vi "ni579x Configure Attenuation.vi"(0 "Register Bus":refnum<class "ni579x Register Bus v1 Host.lvclass">=refnum, 1 "scope":string(combo)="rx/atten1", 5 "attenuation [dB]":dbl format="%#_6p", 11 "Error In":errorcluster) -> (4 "Register Bus (out)":refnum<class "ni579x Register Bus v1 Host.lvclass">, 6 "coerced attenuation [dB]":dbl format="%#_6p", 15 "Error Out":errorcluster)   [LabVIEW 2013]
uses:
  <instrlib>/ni579x/Register Bus/v1/Host/ni579x Register Bus v1 Host.lvclass
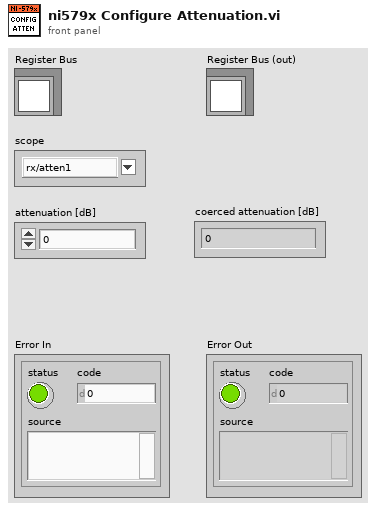
[diagram p1: front panel]
types:
  T1 = typedef "ni579x User Command.ctl" = cluster{"User Data 0":u8, "User Data 1":u8, "User Command ID":T2}
  T2 = typedef "ni579x User Command ID.ctl" = u8
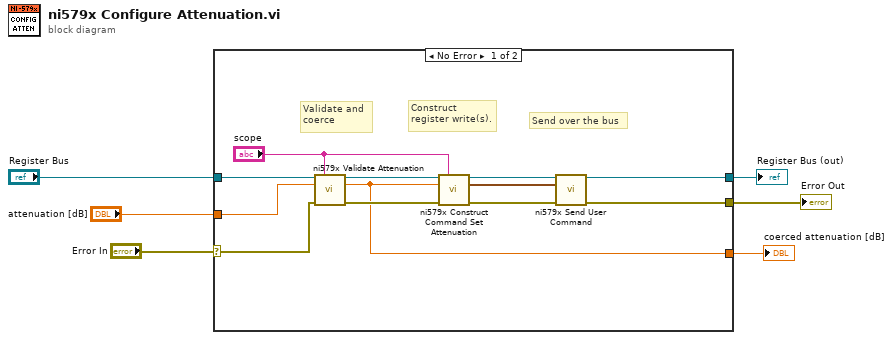
[diagram p0: block diagram]
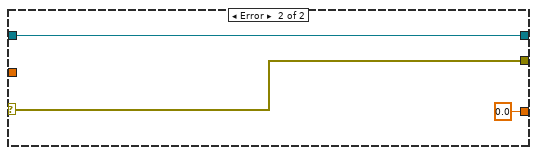
[diagram p2: hidden frame]
diagram:
  n1 = case shown="No Error" "Error In" {
    selector: "Error In" -> [w16 w21]
    tunnel: [w9 w21] -> w5
    tunnel: "Register Bus" -> [w18 w20]
    tunnel: "attenuation [dB]" -> [w17 _]
    tunnel: [w10 w20] -> w2
    tunnel: [w8 0.0 ("coerced attenuation [dB]")] -> w1
    frame No Error {
      # "Send over the bus"
      # "Construct\nregister write(s)."
      # "Validate and \ncoerce"
      n2 = call <instrlib>:"ni579x Validate Attenuation.vi"("Register Bus"=w18, "scope"="scope", "attenuation [dB]"=w17, "Error In"=w16) -> ("Register Bus (out)"=w14:refnum<class "ni579x Register Bus v1 Host.lvclass">, "coerced attenuation [dB]"=w8:dbl, "Error Out"=w15:errorcluster)  [unwired: 9 in]
      n3 = call <instrlib>:"ni579x Construct Command Set Attenuation.vi"("Register Bus"=w14, "scope"="scope", "attenuation [dB]"=w8, "Error In"=w15) -> ("Register Bus (out)"=w12:refnum<class "ni579x Register Bus v1 Host.lvclass">, "User Command"=w7:T1, "Error Out"=w11:errorcluster)  [unwired: 9 in]
      n4 = call <instrlib>:"ni579x Send User Command.vi"("Register Bus"=w12, "User Command"=w7, "Error In"=w11) -> ("Register Bus (out)"=w10:refnum<class "ni579x Register Bus v1 Host.lvclass">, "Error Out"=w9:errorcluster)  [unwired: 8 in, 3 out]
    }
    frame Error {
    }
  }
  "Register Bus (out)" <- w2
  "Error Out" <- w5
  "coerced attenuation [dB]" <- w1
